vi "KMAX close.vi"(8 "error in (no error)":errorcluster, 10 "Image Out":T2, 11 "Refnum in":T1) -> (0 "error out":errorcluster)   [LabVIEW 2023]
uses:
  <vilib>/vision/driver/NI_Vision_Acquisition_Software.lvlib
  <vilib>/vision/Image Controls.llb/IMAQ Image.ctl
  <vilib>/userDefined/High Color/IMAQdx.ctl
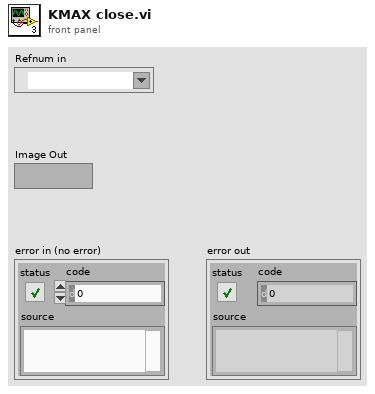
[diagram p1: front panel]
types:
  T1 = typedef "IMAQdx.ctl" = refnum<k21>
  T2 = typedef "IMAQ Image.ctl" = refnum<image>
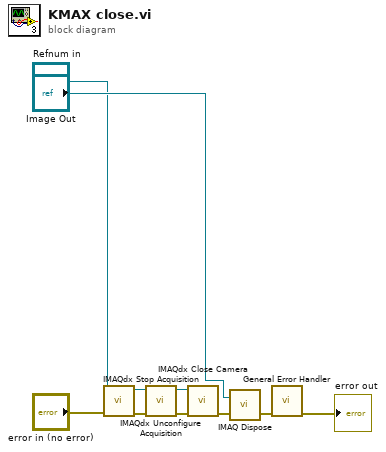
[diagram p0: block diagram]
diagram:
  n1 = call <vilib>:"IMAQdx Stop Acquisition.vi"("error in"="error in (no error)", "Session In"="Refnum in") -> ("error out"=w6:errorcluster, "Session Out"=w5:T1)  [unwired: 8 out]
  n2 = call <vilib>:"IMAQdx Unconfigure Acquisition.vi"("error in"=w6, "Session In"=w5) -> ("error out"=w3:errorcluster, "Session Out"=w4:T1)  [unwired: 8 out]
  n3 = call <vilib>:"IMAQdx Close Camera.vi"("error in"=w3, "Session In"=w4) -> ("error out"=w7:errorcluster)  [unwired: 9 out]
  n4 = call "IMAQ Dispose"("Image"="Image Out", "error in (no error)"=w7) -> ("error out"=w8:errorcluster)  [unwired: 4 in]
  n5 = call <vilib>:"General Error Handler.vi"("error in (no error)"=w8) -> ("error out"=→"error out":errorcluster)  [unwired: 2 in, 12 out]
